vi "PIX2POS.vi"(6 "Table limits":T1, 8 "error in (no error)":errorcluster, 11 "VI Folder Path":path) -> (0 "error out":errorcluster, 2 "C std err":string, 3 "C return":i32)   [LabVIEW 2023]
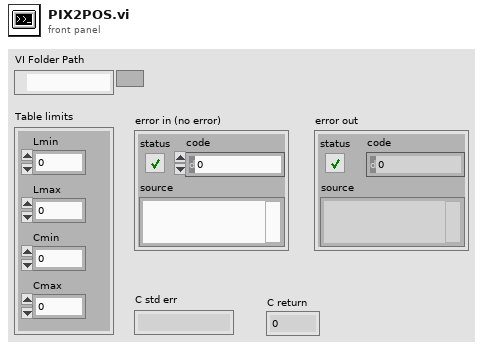
[diagram p1: front panel]
types:
  T1 = cluster{"Lmin":i32, "Lmax":i32, "Cmin":i32, "Cmax":i32}
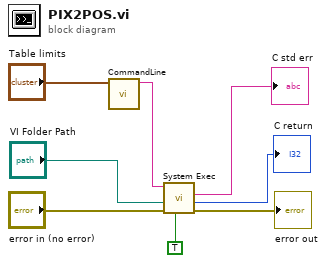
[diagram p0: block diagram]
diagram:
  n1 = call "CommandLine.vi"("Table limits"="Table limits") -> ("Command line"=w1:string)  [unwired: 10 in]
  n2 = call <vilib>:"System Exec.vi"("run minimized? (F)"=TRUE, "error in (no error)"="error in (no error)", "working directory"="VI Folder Path", "command line"=w1) -> ("error out"=→"error out":errorcluster, "return code"=→"C return":i32, "standard error"=→"C std err":string)  [unwired: 4 in, 1 out]
